vi "Three Button Dialog CORE.vi"(4 "Allow user to close window? (TRUE)":bool=TRUE, 5 "Justify Message (Left)":enum16{"Left", "Center", "Right"}(ring), 6 "Keyboard Shortcuts (Left is <Enter>)":T1={"Left Button Key Shortcut"={"Control"=FALSE, "Shift"=FALSE, "Key"="<Enter>"}, "Center Button Key Shortcut"={"Control"=FALSE, "Shift"=FALSE, "Key"=""}, "Right Button Key Shortcut"={"Control"=FALSE, "Shift"=FALSE, "Key"=""}}, 7 "Window Title (\"\")":string, 8 "Right Button Text (\"Cancel\")":string="Cancel", 9 "Center Button Text (\"No\")":string="No", 10 "Left Button Text (\"Yes\")":string="Yes", 11 "message":string) -> (3 "Which Button?":T2(ring)=enum."Center Button")   [LabVIEW 2015]
doc: "Displays text in a dialog with three buttons. The output enum indicates which of the three buttons the user chose, or it indicates that the user closed the dialog without making any choice."
uses:
  miscctls.llb/LVRectTypeDef.ctl
panel:
  in  "OK":string="OK"
  out "C-Message":string
  in  "Right Button":bool
  in  "Center Button":bool
  in  "Left Button":bool
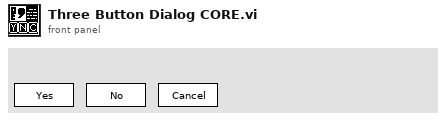
[diagram p1: front panel]
types:
  T1 = cluster{"Left Button Key Shortcut":cluster{"Control":bool, "Shift":bool, "Key":string}, "Center Button Key Shortcut":cluster{"Control":bool, "Shift":bool, "Key":string}, "Right Button Key Shortcut":cluster{"Control":bool, "Shift":bool, "Key":string}}
  T2 = enum16{"Left Button", "Center Button", "Right Button", "Window Close"}
  T3 = cluster{"left":i16, "top":i16, "right":i16, "bottom":i16}
  T4 = cluster{"Control":bool, "Shift":bool, "Key":string}
  T5 = cluster{bool, "Control":bool, "Shift":bool, "Key":string}
  T6 = typedef "LVRectTypeDef.ctl" = cluster{"Left":i16, "Top":i16, "Right":i16, "Bottom":i16}
  T7 = typedef "LVBoundsTypeDef.ctl" = cluster{"Width":u32, "Height":u32}
  T8 = typedef "LVPointTypeDef.ctl" = cluster{"Horizontal":i16, "Vertical":i16}
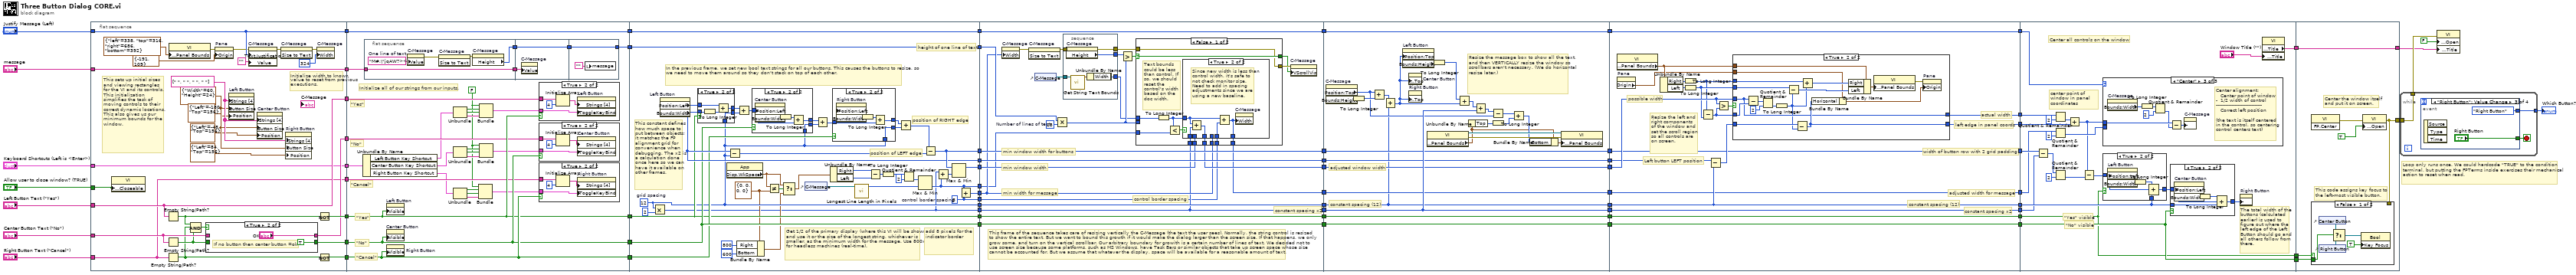
[diagram p0: block diagram]
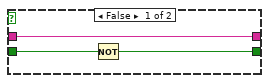
[diagram p2: hidden frame]
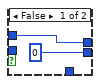
[diagram p6: hidden frame]
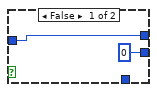
[diagram p7: hidden frame]
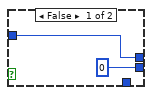
[diagram p8: hidden frame]
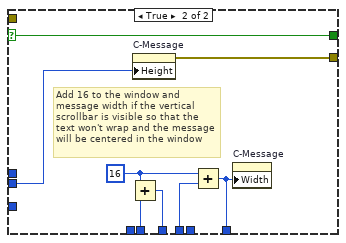
[diagram p10: hidden frame]
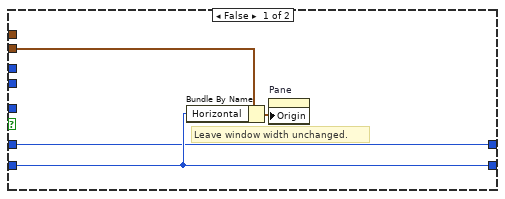
[diagram p11: hidden frame]
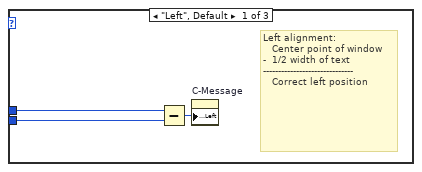
[diagram p12: hidden frame]
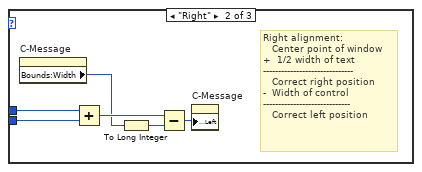
[diagram p13: hidden frame]
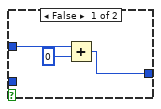
[diagram p14: hidden frame]
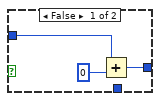
[diagram p15: hidden frame]
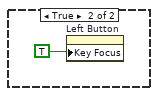
[diagram p16: hidden frame]
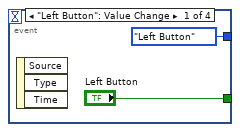
[diagram p17: hidden frame]
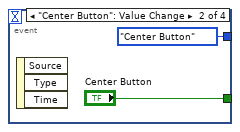
[diagram p18: hidden frame]
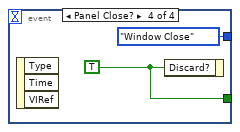
[diagram p19: hidden frame]
diagram:
  # "Loop only runs once. We could hardcode \"TRUE\" to the condition terminal, but putting the FPTerms inside exercises their mechanical action to reset when read."
  n1 = flat-sequence {
    tunnel: [w86] -> w14
    tunnel: [w88] -> w13
    tunnel: [w87] -> w12
    tunnel: [w82] -> w11
    tunnel: [w83] -> w10
    tunnel: [w80] -> w9
    tunnel: [w79] -> w8
    tunnel: "Left Button Text (\"Yes\")" -> [w82]
    tunnel: "Center Button Text (\"No\")" -> [w81]
    tunnel: "Right Button Text (\"Cancel\")" -> [w80]
    tunnel: "Justify Message (Left)" -> [w79]
    tunnel: "Keyboard Shortcuts (Left is <Enter>)" -> [w76]
    tunnel: [w76] -> w7
    tunnel: "message" -> [w75]
    tunnel: [w75] -> w6
    tunnel: "Allow user to close window? (TRUE)" -> [w74]
    tunnel: w14 -> [w130]
    tunnel: [w130] -> w64
    tunnel: w13 -> [w129]
    tunnel: [w129] -> w63
    tunnel: w12 -> [w128]
    tunnel: [w128] -> w62
    tunnel: w11 -> [w127]
    tunnel: w10 -> [w126]
    tunnel: w9 -> [w125]
    tunnel: w8 -> [w124]
    tunnel: [w124] -> w61
    tunnel: [w120] -> w60
    tunnel: w7 -> [w123]
    tunnel: w6 -> [w119]
    tunnel: [w191] -> w59
    tunnel: [w188] -> w58
    tunnel: [w187] -> w57
    tunnel: [w170] -> w56
    tunnel: [w152] -> w55
    tunnel: w64 -> [w180]
    tunnel: w63 -> [w182]
    tunnel: [w182] -> w54
    tunnel: w62 -> [w178]
    tunnel: [w178] -> w53
    tunnel: [w163] -> w52
    tunnel: w61 -> [w173]
    tunnel: [w173] -> w51
    tunnel: w60 -> [w172]
    tunnel: [w172] -> w50
    tunnel: [w161] -> w3
    tunnel: [w160] -> w2
    tunnel: w59 -> [w226]
    tunnel: [w225] -> w49
    tunnel: w58 -> [w232]
    tunnel: [w232] -> w48
    tunnel: w57 -> [w231]
    tunnel: [w231] -> w47
    tunnel: w56 -> [w230]
    tunnel: [w230] -> w46
    tunnel: w55 -> [w219]
    tunnel: [w219] -> w45
    tunnel: w54 -> [w229]
    tunnel: [w229] -> w44
    tunnel: w53 -> [w228]
    tunnel: [w228] -> w43
    tunnel: w52 -> [w220]
    tunnel: [w224] -> w42
    tunnel: w51 -> [w227]
    tunnel: [w227] -> w41
    tunnel: w50 -> [w222]
    tunnel: w3 -> [w218]
    tunnel: w2 -> [w217]
    tunnel: w49 -> [w281]
    tunnel: [w281] -> w40
    tunnel: w48 -> [w280]
    tunnel: [w280] -> w39
    tunnel: w47 -> [w279]
    tunnel: [w279] -> w38
    tunnel: w46 -> [w272]
    tunnel: [w272] -> w37
    tunnel: w45 -> [w289]
    tunnel: [w289] -> w36
    tunnel: w44 -> [w278]
    tunnel: [w278] -> w35
    tunnel: w43 -> [w277]
    tunnel: [w277] -> w34
    tunnel: w42 -> [w276]
    tunnel: [w276] -> w33
    tunnel: w41 -> [w275]
    tunnel: [w275] -> w32
    tunnel: w40 -> [w316]
    tunnel: [w311] -> w31
    tunnel: w39 -> [w304]
    tunnel: [w304] -> w30
    tunnel: w38 -> [w310]
    tunnel: w37 -> [w309]
    tunnel: [w309] -> w29
    tunnel: w36 -> [w303]
    tunnel: [w303] -> w28
    tunnel: [w307] -> w27
    tunnel: w35 -> [w302]
    tunnel: [w302] -> w26
    tunnel: w34 -> [w301]
    tunnel: [w301] -> w25
    tunnel: w33 -> [w298]
    tunnel: [w298] -> w24
    tunnel: w32 -> [w300]
    tunnel: [w300] -> w23
    tunnel: [w341] -> w22
    tunnel: w31 -> [w360]
    tunnel: w30 -> [w353]
    tunnel: w29 -> [w357]
    tunnel: w28 -> [w352]
    tunnel: w27 -> [w359]
    tunnel: w26 -> [w340]
    tunnel: w25 -> [w339]
    tunnel: w24 -> [w345]
    tunnel: w23 -> [w346]
    tunnel: [w340] -> w5
    tunnel: [w339] -> w4
    tunnel: [w394] -> w67
    tunnel: [w396] -> w65
    tunnel: w22 -> [w396]
    tunnel: w5 -> [w392]
    tunnel: w4 -> [w393]
    frame #0 {
      w96 = string[] [" ", " ", " ", " "] ("Strings [4]")
      w95 = cluster{"Width":u32, "Height":u32} {"Width"=60, "Height"=24} ("Button Size")
      # "Initialize width to known value to reset from previous executions."
      # "This sets up initial sizes and viewing rectangles\nfor the VI and its controls. This initialization\nsimplifies the task of moving controls to their\ncorrect dynamic locations. This also gives us our\nminimum bounds for the window."
      n2 = property class="VI"("Front Panel Window:Closeable"=w74) -> ()  [unwired: 2 in, 2 out]
      n3 = Empty String/Path?(string/path=w82) -> (empty?=w90:bool)
      n4 = Empty String/Path?(string/path=w81) -> (empty?=w78:bool)
      n5 = Empty String/Path?(string/path=w80) -> (empty?=w77:bool)
      n6 = property class="VI"("Front Panel Window:Panel Bounds"=T3 {"left"=338, "top"=316, "right"=686, "bottom"=392} ("Front Panel.PanelBounds")) -> (error out=w73:errorcluster)  [unwired: 2 in, 1 out]
      n7 = Compound Arithmetic op=AND(w90, w77, w78) -> (w89:bool)
      n8 = case shown="True" w89 {
        tunnel: w78 -> [w99 _]
        tunnel: [w98 TRUE] -> w88
        tunnel: w81 -> [w97 _]
        tunnel: [w97 "OK"] -> w83
        frame False {
          n9 = Not(x=w99) -> (.not. x?=w98:bool)
        }
        frame True {
          # "If no button then center button =ok"
        }
      }
      n10 = property on="Pane" class="Pane"(error in=w73, "Origin"=cluster{"Horizontal":i16, "Vertical":i16} {"Horizontal"=-191, "Vertical"=109} ("Front Panel.Origin")) -> (error out=w72:errorcluster)  [unwired: 1 in, 1 out]
      n11 = property on="Left Button" class="Bool"("Strings [4]"=w96, "Button Size"=w95, "Position"=cluster{"Left":i32, "Top":i32} {"Left"=-180, "Top"=156}) -> ()  [unwired: 2 in, 2 out]
      n12 = property on="C-Message" class="Str"(error in=w72, "Text.Justification"=w79, "Value"="") -> (error out=w91:errorcluster)  [unwired: 1 in, 1 out]
      n13 = property on="Center Button" class="Bool"("Strings [4]"=w96, "Button Size"=w95, "Position"=cluster{"Left":i32, "Top":i32} {"Left"=-48, "Top"=156}) -> ()  [unwired: 2 in, 2 out]
      n14 = invoke on="C-Message" class="Str" method="Size to Text"(error in=w91) -> (error out=w70:errorcluster)  [unwired: 2 in, 2 out]
      n15 = property on="Right Button" class="Bool"("Strings [4]"=w96, "Button Size"=w95, "Position"=cluster{"Left":i32, "Top":i32} {"Left"=84, "Top"=156}) -> ()  [unwired: 2 in, 2 out]
      n16 = property on="C-Message" class="Str"(error in=w70, "Width"=u32 324 ("Size:Width")) -> ()  [unwired: 1 in, 2 out]
      n17 = Not(x=w90) -> (.not. x?=w87:bool)
      n18 = Not(x=w77) -> (.not. x?=w86:bool)
    }
    frame #1 {
      w104 = FALSE
      # "\"Cancel\""
      # "\"No\""
      # "\"Yes\""
      # "\"Cancel\""
      # "\"No\""
      # "\"Yes\""
      # "Initialize all of our strings from our inputs."
      n19 = Unbundle By Name(w123) -> ("Left Button Key Shortcut"=w117:T4, "Center Button Key Shortcut"=w109:T4, "Right Button Key Shortcut"=w103:T4)
      n20 = flat-sequence {
        tunnel: [w132] -> w122
        tunnel: w119 -> [w131]
        tunnel: [w131] -> w118
        tunnel: w122 -> [w137]
        tunnel: [w137] -> w121
        tunnel: w118 -> [w136]
        tunnel: w121 -> [w138]
        tunnel: [w138] -> w120
        frame #0 {
          w135 = "M#,\"jqAW?><"  # One line of text
          n21 = property on="C-Message" class="Str"("Value"=w135) -> (error out=w133:errorcluster)  [unwired: 2 in, 1 out]
          n22 = invoke on="C-Message" class="Str" method="Size to Text"(error in=w133) -> (error out=w134:errorcluster)  [unwired: 2 in, 2 out]
          n23 = property on="C-Message" class="Str"(error in=w134) -> ("Height"=w132:u32)  [unwired: 1 in, 2 out]
        }
        frame #1 {
          n24 = property on="C-Message" class="Str"("Value"=w136) -> ()  [unwired: 2 in, 2 out]
        }
        frame #2 {
          n25 = local write "message"("") -> ()
        }
      }
      n26 = property on="Left Button" class="Bool"("Visible"=w128) -> ()  [unwired: 2 in, 2 out]
      n27 = property on="Center Button" class="Bool"("Visible"=w129) -> ()  [unwired: 2 in, 2 out]
      n28 = property on="Right Button" class="Bool"("Visible"=w130) -> ()  [unwired: 2 in, 2 out]
      n29 = Unbundle(w117) -> ("Control"=w116:bool, "Shift"=w115:bool, "Key"=w114:string)
      n30 = Unbundle(w109) -> ("Control"=w112:bool, "Shift"=w111:bool, "Key"=w110:string)
      n31 = Unbundle(w103) -> ("Control"=w107:bool, "Shift"=w106:bool, "Key"=w105:string)
      n32 = Bundle(w104, "Control"=w107, "Shift"=w106, "Key"=w105) -> (w102:T5)  [unwired: 1 in]
      n33 = Bundle(w104, "Control"=w116, "Shift"=w115, "Key"=w114) -> (w113:T5)  [unwired: 1 in]
      n34 = Bundle(w104, "Control"=w112, "Shift"=w111, "Key"=w110) -> (w108:T5)  [unwired: 1 in]
      n35 = case shown="True" w128 {
        tunnel: w127 -> [_ w149]
        tunnel: w113 -> [_ w148]
        frame False {
        }
        frame True {
          n36 = Initialize Array(w149, 4 ("dimension size")) -> (w151:string[])
          n37 = property on="Left Button" class="Bool"("Strings [4]"=w151, "ToggleKeyBind"=w148) -> ()  [unwired: 2 in, 2 out]
        }
      }
      n38 = case shown="True" w129 {
        tunnel: w108 -> [_ w145]
        tunnel: w126 -> [_ w144]
        frame False {
        }
        frame True {
          n39 = Initialize Array(w144, 4 ("dimension size")) -> (w147:string[])
          n40 = property on="Center Button" class="Bool"("Strings [4]"=w147, "ToggleKeyBind"=w145) -> ()  [unwired: 2 in, 2 out]
        }
      }
      n41 = case shown="True" w130 {
        tunnel: w102 -> [_ w141]
        tunnel: w125 -> [_ w140]
        frame False {
        }
        frame True {
          n42 = Initialize Array(w140, 4 ("dimension size")) -> (w143:string[])
          n43 = property on="Right Button" class="Bool"("Strings [4]"=w143, "ToggleKeyBind"=w141) -> ()  [unwired: 2 in, 2 out]
        }
      }
    }
    frame #2 {
      w157 = T6 {"Left"=0, "Top"=0, "Right"=0, "Bottom"=0} ("Display:Primary Workspace")
      w161 = 8  # control border spacing
      w170 = 12  # grid spacing
      # "position of RIGHT edge"
      # "height of one line of text"
      # "add 8 pixels for the indicator border"
      # "Get 1/2 of the primary display (where this VI will be shown) and use it or the size of the longest string, whichever is smaller, as the minimum width for the message. Use 800x600 for headless machines (real-time)."
      # "This constant defines how much space to put between objects; it matches the FP alignment grid for convenience when debugging. The x2 is a calculation done once here so we can have it available on other frames."
      # "In the previous frame, we set new bool text strings for all our buttons. This causes the buttons to resize, so we need to move them around so they don't stack on top of each other."
      # "position of LEFT edge"
      n44 = Multiply(x=w170, y=2) -> (x*y=w152:i32)
      n45 = property on="Left Button" class="Bool"() -> ("Position:Left"=w187:i32, "Bounds:Width"=w184:u32)  [unwired: 2 in, 2 out]
      n46 = case shown="True" w178 {
        tunnel: w187 -> [w194 w199]
        tunnel: w184 -> [_ w198]
        tunnel: [w194 w197] -> w179
        tunnel: w170 -> [_ w195]
        tunnel: [0 w195] -> w177
        frame False {
        }
        frame True {
          n47 = To Long Integer(number=w198) -> (32bit integer=w196:i32)
          n48 = Add(x=w199, y=w196) -> (x+y=w197:i32)
        }
      }
      n49 = property class="App"() -> ("Disp.WkSpace"=w158:T6)  [unwired: 2 in, 2 out]
      n50 = Subtract(x=w187, y=w170) -> (x-y=w189:i32)
      n51 = Bundle By Name(cluster=w157, "Right"=i16 800, "Bottom"=i16 600) -> (w154:T6)
      n52 = Add(x=w179, y=w177) -> (x+y=w185:i32)
      n53 = case shown="True" w182 {
        tunnel: w185 -> [w208 w213]
        tunnel: [w208 w212] -> w183
        tunnel: [0 w209] -> w176
        tunnel: w170 -> [_ w209]
        frame False {
        }
        frame True {
          n54 = property on="Center Button" class="Bool"("Position:Left"=w213) -> ("Bounds:Width"=w211:u32)  [unwired: 2 in, 2 out]
          n55 = To Long Integer(number=w211) -> (32bit integer=w210:i32)
          n56 = Add(x=w210, y=w213) -> (x+y=w212:i32)
        }
      }
      n57 = Not Equal?(x=w158, y=w157) -> (x != y?=w159:bool)
      n58 = Select(t=w158, s=w159, f=w154) -> (s? t:f=w153:T6)
      n59 = control-ref of="C-Message"() -> (w174:refnum<vi>)
      n60 = Add(x=w183, y=w176) -> (x+y=w186:i32)
      n61 = Unbundle By Name(w153) -> ("Right"=w166:i16, "Left"=w165:i16)
      n62 = case shown="True" w180 {
        tunnel: w186 -> [w201 w206]
        tunnel: [w201 w202] -> w181
        tunnel: [0 w203] -> w175
        tunnel: w170 -> [_ w203]
        frame False {
        }
        frame True {
          n63 = property on="Right Button" class="Bool"("Position:Left"=w206) -> ("Bounds:Width"=w205:u32)  [unwired: 2 in, 2 out]
          n64 = To Long Integer(number=w205) -> (32bit integer=w204:i32)
          n65 = Add(x=w204, y=w206) -> (x+y=w202:i32)
        }
      }
      n66 = call "Longest Line Length in Pixels.vi"("String"=w174) -> ("longest line length"=w167:i32)  [unwired: 9 in]
      n67 = Subtract(x=w166, y=w165) -> (x-y=w169:i16)
      n68 = To Long Integer(number=w169) -> (32bit integer=w164:i32)
      n69 = Add(x=w181, y=w175) -> (x+y=w190:i32)
      n70 = Quotient & Remainder(x=w164, y=2) -> (floor(x/y)=w162:i32)  [unwired: 1 out]
      n71 = Max & Min(x=w162, y=w167) -> (min(x,y)=w160:i32)  [unwired: 1 out]
      n72 = Subtract(x=w190, y=w189) -> (x-y=w188:i32)
      n73 = Add(x=w152, y=w160) -> (x+y=w192:i32)
      n74 = Max & Min(x=w188, y=w192) -> (max(x,y)=w191:i32)  [unwired: 1 out]
      n75 = Add(x=w160, y=w161) -> (x+y=w163:i32)
    }
    frame #3 {
      w234 = u32 25  # Number of lines of text
      # "control border spacing"
      # "constant spacing x2"
      # "min window width for buttons"
      # "min window width"
      # "min width for message"
      # "This frame of the sequence takes care of resizing vertically the C-Message (the text the user sees). Normally, the string control is resized to show the entire text. But we want to bound this growth if it would make the dialog larger than the screen size. If that happens, we only grow some, and turn on the vertical scrollbar. Our arbitrary boundary for growith is a certain number of lines of text. We decided not to use screen size because some platforms, such as MS Windows, have Task Bars or similar objects that take up screen space whose size cannot be accounted for. But we assume that whatever the display, space will be available for a reasonable amount of text."
      n76 = property on="C-Message" class="Str"("Width"=w220) -> (error out=w223:errorcluster)  [unwired: 2 in, 1 out]
      n77 = invoke on="C-Message" class="Str" method="Size to Text"(error in=w223) -> (error out=w238:errorcluster)  [unwired: 2 in, 2 out]
      n78 = control-ref of="C-Message"() -> (w215:refnum<vi>)
      n79 = Multiply(x=w222, y=w234) -> (x*y=w233:u32)
      n80 = stacked-sequence {
        tunnel: w238 -> [w244]
        tunnel: [w243] -> w221
        tunnel: [w242] -> w216
        tunnel: w215 -> [w241]
        tunnel: [w239] -> w214
        frame #0 {
          n81 = property on="C-Message" class="Str"(error in=w244) -> (error out=w242:errorcluster, "Height"=w243:u32)  [unwired: 1 in, 1 out]
          n82 = call "Get String Text Bounds.vi"("String"=w241) -> ("Text bounds"=w240:T7)  [unwired: 10 in]
          n83 = Unbundle By Name(w240) -> ("Width"=w239:u32)
        }
      }
      n84 = Greater?(x=w221, y=w233) -> (0:w237:bool)
      n85 = case shown="False" w237 {
        selector: w237 -> [w256 w270]
        tunnel: [w255 w271] -> w236
        tunnel: [w256 w270] -> w235
        tunnel: w216 -> [w255 _]
        tunnel: w233 -> [_ w269]
        tunnel: [w249 w267] -> w225
        tunnel: w226 -> [w251 w268]
        tunnel: [w248 w264] -> w224
        tunnel: w220 -> [w250 w266]
        tunnel: w214 -> [w253 _]
        tunnel: w217 -> [w252 _]
        tunnel: w219 -> [w247 _]
        tunnel: w218 -> [w246 _]
        frame False {
          # "Text bounds could be less than control. If so, we should reset the control's width based on the doc width."
          n86 = To Long Integer(number=w253) -> (32bit integer=w245:i32)
          n87 = Less?(x=w245, y=w252) -> (x < y?=w254:bool)
          n88 = case shown="True" w254 {
            tunnel: w245 -> [_ w262]
            tunnel: w251 -> [w258 _]
            tunnel: w250 -> [w257 _]
            tunnel: [w258 w261] -> w249
            tunnel: [w257 w260] -> w248
            tunnel: w247 -> [_ w263]
            tunnel: w246 -> [_ w259]
            frame False {
            }
            frame True {
              # "Since new width is less than control width, it's safe to not check monitor size. \nNeed to add in spacing adjustments since we are using a new baseline."
              n89 = Add(x=w262, y=w263) -> (x+y=w261:i32)
              n90 = Add(x=w262, y=w259) -> (x+y=w260:i32)
              n91 = property on="C-Message" class="Str"("Width"=w260) -> ()  [unwired: 2 in, 2 out]
            }
          }
        }
        frame True {
          w265 = 16 ("x")
          # "Add 16 to the window and message width if the vertical scrollbar is visible so that the text won't wrap and the message will be centered in the window"
          n92 = Add(x=w265, y=w268) -> (x+y=w267:i32)
          n93 = property on="C-Message" class="Str"("Height"=w269) -> (error out=w271:errorcluster)  [unwired: 2 in, 1 out]
          n94 = Add(x=w265, y=w266) -> (x+y=w264:i32)
          n95 = property on="C-Message" class="Str"("Width"=w264) -> ()  [unwired: 2 in, 2 out]
        }
      }
      n96 = property on="C-Message" class="Str"(error in=w236, "VScrollVis"=w235) -> ()  [unwired: 1 in, 2 out]
    }
    frame #4 {
      # "adjusted window width"
      # "constant spacing (12)"
      # "Resize the message box to show all the text, and then VERTICALLY resize the window so scrollbars aren't necessary. (We do horizontal resize later.)"
      n97 = property on="C-Message" class="Str"() -> ("Position:Top"=w283:i32, "Bounds:Height"=w282:u32)  [unwired: 2 in, 2 out]
      n98 = To Long Integer(number=w282) -> (32bit integer=w288:i32)
      n99 = Add(x=w283, y=w288) -> (x+y=w273:i32)
      n100 = Add(x=w273, y=w272) -> (x+y=w274:i32)
      n101 = property on="Left Button" class="Bool"("Position:Top"=w274) -> ("Bounds:Height"=w285:u32)  [unwired: 2 in, 2 out]
      n102 = property on="Center Button" class="Bool"("Position:Top"=w274) -> ()  [unwired: 2 in, 2 out]
      n103 = property on="Right Button" class="Bool"("Position:Top"=w274) -> ()  [unwired: 2 in, 2 out]
      n104 = property class="VI"() -> (reference out=w295:refnum<vi>, error out=w296:errorcluster, "Front Panel Window:Panel Bounds"=w286:T6)  [unwired: 2 in]
      n105 = To Long Integer(number=w285) -> (32bit integer=w284:i32)
      n106 = Add(x=w284, y=w274) -> (x+y=w290:i32)
      n107 = Unbundle By Name(w286) -> ("Top"=w293:i16)
      n108 = Add(x=w290, y=w289) -> (x+y=w291:i32)
      n109 = Subtract(x=w291, y=w283) -> (x-y=w294:i32)
      n110 = To Long Integer(number=w293) -> (32bit integer=w287:i32)
      n111 = Add(x=w294, y=w287) -> (x+y=w292:i32)
      n112 = Bundle By Name(cluster=w286, "Bottom"=w292) -> (w297:T6)
      n113 = property class="VI"(reference=w295, error in=w296, "Front Panel Window:Panel Bounds"=w297) -> ()  [unwired: 2 out]
    }
    frame #5 {
      # "adjusted width for message"
      # "constant spacing x2"
      # "constant spacing (12)"
      # "Left button LEFT position"
      # "left edge in panel coords"
      # "width of button row with 2 grid padding"
      # "Resize the left and\nright components\nof the window and\nset the scroll region\nso all controls are \non screen."
      # "actual width"
      # "possible width"
      n114 = property class="VI"() -> ("Front Panel Window:Panel Bounds"=w313:T6)  [unwired: 2 in, 2 out]
      n115 = property on="Pane" class="Pane"() -> ("Origin"=w299:T8)  [unwired: 2 in, 2 out]
      n116 = Unbundle By Name(w313) -> ("Right"=w315:i16, "Left"=w314:i16)
      n117 = To Long Integer(number=w315) -> (32bit integer=w305:i32)
      n118 = To Long Integer(number=w314) -> (32bit integer=w306:i32)
      n119 = Subtract(x=w305, y=w306) -> (x-y=w317:i32)
      n120 = Subtract(x=w310, y=w309) -> (x-y=w308:i32)
      n121 = Greater?(x=w316, y=w317) -> (0:w312:bool)
      n122 = case shown="True" w312 {
        tunnel: w317 -> [w319 w338]
        tunnel: w316 -> [_ w325]
        tunnel: w305 -> [_ w333]
        tunnel: w306 -> [_ w334]
        tunnel: w313 -> [_ w335]
        tunnel: [w321 w327] -> w311
        tunnel: w299 -> [w320 w328]
        tunnel: w308 -> [w321 w326]
        tunnel: [w319 w325] -> w307
        frame False {
          # "Leave window width unchanged."
          n123 = Bundle By Name(cluster=w320, "Horizontal"=w321) -> (w318:T8)
          n124 = property on="Pane" class="Pane"("Origin"=w318) -> ()  [unwired: 2 in, 2 out]
        }
        frame True {
          n125 = Subtract(x=w325, y=w338) -> (x-y=w337:i32)
          n126 = Quotient & Remainder(x=w337, y=2) -> (floor(x/y)=w330:i32)  [unwired: 1 out]
          n127 = To Long Integer(number=w330) -> (32bit integer=w324:i32)
          n128 = Subtract(x=w334, y=w324) -> (x-y=w331:i32)
          n129 = Subtract(x=w326, y=w324) -> (x-y=w327:i32)
          n130 = Add(x=w333, y=w324) -> (x+y=w332:i32)
          n131 = Bundle By Name(cluster=w328, "Horizontal"=w327) -> (w322:T8)
          n132 = Bundle By Name(cluster=w335, "Right"=w332, "Left"=w331) -> (w329:T6)
          n133 = property class="VI"("Front Panel Window:Panel Bounds"=w329) -> (error out=w323:errorcluster)  [unwired: 2 in, 1 out]
          n134 = property on="Pane" class="Pane"(error in=w323, "Origin"=w322) -> ()  [unwired: 1 in, 2 out]
        }
      }
    }
    frame #6 {
      # "\"No\" visible"
      # "\"Yes\" visible"
      # "The total width of the buttons (calculated earlier) is used to figure out where the left edge of the Left Button should go and all others follow from there."
      # "center point of window in panel coordinates"
      # "Center all controls on the window"
      n135 = Subtract(x=w353, y=w352) -> (x-y=w354:i32)
      n136 = Quotient & Remainder(x=w359, y=2) -> (floor(x/y)=w356:i32)  [unwired: 1 out]
      n137 = Quotient & Remainder(x=w345, y=2) -> (floor(x/y)=w344:i32)  [unwired: 1 out]
      n138 = Quotient & Remainder(x=w354, y=2) -> (floor(x/y)=w351:i32)  [unwired: 1 out]
      n139 = Add(x=w356, y=w360) -> (x+y=w343:i32)
      n140 = Subtract(x=w343, y=w351) -> (x-y=w350:i32)
      n141 = case shown="\"Center\"" w346 {
        tunnel: w343 -> [w363 w369 w371]
        tunnel: w344 -> [w361 w368 _]
        frame "Left", Default {
          # "Left alignment:\n   Center point of window\n-  1/2 width of text\n------------------------------\n   Correct left position"
          n142 = Subtract(x=w363, y=w361) -> (x-y=w362:i32)
          n143 = property on="C-Message" class="Str"("Position:Left"=w362) -> ()  [unwired: 2 in, 2 out]
        }
        frame "Right" {
          # "Right alignment:\n   Center point of window\n+  1/2 width of text\n------------------------------\n   Correct right position\n-  Width of control\n-----------------------------\n   Correct left position"
          n144 = property on="C-Message" class="Str"() -> ("Bounds:Width"=w365:u32)  [unwired: 2 in, 2 out]
          n145 = Add(x=w369, y=w368) -> (x+y=w367:i32)
          n146 = To Long Integer(number=w365) -> (32bit integer=w364:i32)
          n147 = Subtract(x=w367, y=w364) -> (x-y=w366:i32)
          n148 = property on="C-Message" class="Str"("Position:Left"=w366) -> ()  [unwired: 2 in, 2 out]
        }
        frame "Center" {
          # "Center alignment:\n   Center point of window\n-  1/2 width of control\n------------------------------\n   Correct left position\n\n(the text is itself centered in the control, so centering control centers text)"
          n149 = property on="C-Message" class="Str"() -> ("Bounds:Width"=w374:u32)  [unwired: 2 in, 2 out]
          n150 = To Long Integer(number=w374) -> (32bit integer=w372:i32)
          n151 = Quotient & Remainder(x=w372, y=2) -> (floor(x/y)=w370:i32)  [unwired: 1 out]
          n152 = Subtract(x=w371, y=w370) -> (x-y=w373:i32)
          n153 = property on="C-Message" class="Str"("Position:Left"=w373) -> ()  [unwired: 2 in, 2 out]
        }
      }
      n154 = case shown="True" w339 {
        tunnel: w357 -> [_ w391]
        tunnel: w350 -> [w386 w390]
        tunnel: [w385 w388] -> w349
        frame False {
          n155 = Add(x=w386, y=0) -> (x+y=w385:i32)
        }
        frame True {
          n156 = property on="Left Button" class="Bool"("Position:Left"=w390) -> ("Bounds:Width"=w389:u32)  [unwired: 2 in, 2 out]
          n157 = To Long Integer(number=w389) -> (32bit integer=w387:i32)
          n158 = Compound Arithmetic op=ADD(w387, w390, w391) -> (w388:i32)
        }
      }
      n159 = case shown="True" w340 {
        tunnel: w357 -> [_ w383]
        tunnel: w349 -> [w378 w381]
        tunnel: [w377 w380] -> w348
        frame False {
          n160 = Add(x=w378, y=0) -> (x+y=w377:i32)
        }
        frame True {
          n161 = property on="Center Button" class="Bool"("Position:Left"=w381) -> ("Bounds:Width"=w382:u32)  [unwired: 2 in, 2 out]
          n162 = To Long Integer(number=w382) -> (32bit integer=w379:i32)
          n163 = Compound Arithmetic op=ADD(w379, w381, w383) -> (w380:i32)
        }
      }
      n164 = property on="Right Button" class="Bool"("Position:Left"=w348) -> ()  [unwired: 2 in, 2 out]
      n165 = property class="VI"("Front Panel Window:Title"="Window Title (\"\")") -> ("Front Panel Window:Title"=w341:string)  [unwired: 2 in, 2 out]
    }
    frame #7 {
      # "This code assigns key focus to\nthe left-most visible button."
      # "Center the window itself and put it on screen."
      n166 = invoke class="VI" method="FP.Center"() -> (error out=w395:errorcluster)  [unwired: 3 in, 2 out]
      n167 = property class="VI"(error in=w395, "Front Panel Window:Open"=TRUE) -> (error out=w394:errorcluster)  [unwired: 1 in, 1 out]
      n168 = case shown="False" w393 {
        tunnel: w394 -> [_ _]
        tunnel: w392 -> [w402 _]
        frame False {
          n169 = control-ref of="Center Button"() -> (w401:refnum<vi>)
          n170 = control-ref of="Right Button"() -> (w400:refnum<vi>)
          n171 = Select(t=w401, s=w402, f=w400) -> (s? t:f=w399:refnum<vi>)
          n172 = property class="Bool"(reference=w399, "Key Focus"=TRUE) -> ()  [unwired: 1 in, 2 out]
        }
        frame True {
          n173 = property on="Left Button" class="Bool"("Key Focus"=TRUE) -> ()  [unwired: 2 in, 2 out]
        }
      }
    }
  }
  n174 = while {
    tunnel: [w406] -> w68
    tunnel: [w405] -> w66
    tunnel: w67 -> [w405]
    stop <- w404 stop-if-true
    n175 = event shown="[2] \"Right Button\": Value Change" {
      selector: _ -> [_ _ _ _]
      dyn-events: _ -> [_ _ _ _]
      timeout: _ -> [_ _ _ _]
      tunnel: ["Left Button" "Center Button" "Right Button" w413] -> w404
      tunnel: [T2."Left Button" ("Which Button?") T2."Center Button" ("Which Button?") T2."Right Button" ("Which Button?") T2."Window Close" ("Which Button?")] -> w406
      event "Left Button": Value Change {
        n176 = event-data() -> ()  [unwired: 1 in, 3 out]
      }
      event "Center Button": Value Change {
        n177 = event-data() -> ()  [unwired: 1 in, 3 out]
      }
      event "Right Button": Value Change {
        n178 = event-data() -> ()  [unwired: 1 in, 3 out]
      }
      event Panel Close? {
        w413 = TRUE ("Discard?")
        n179 = event-data() -> ()  [unwired: 1 in, 3 out]
        n180 = event-data("Discard?"=w413) -> ()  [unwired: 1 in, 1 out]
      }
    }
  }
  "Which Button?" <- w68
  n181 = property class="VI"(error in=w66, "Front Panel Window:Open"=FALSE, "Front Panel Window:Title"=w65) -> ()  [unwired: 1 in, 2 out]
